vi "Dashboard Main.vi"() -> ()   [LabVIEW 2020]
uses:
  <vilib>/Utility/miscctls.llb/LVRowAndColumnTypeDef.ctl
  <vilib>/event_ctls.llb/eventvkey.ctl
  d97281b5-a6a5-4d38-a890-f2f672331580.vi
  <vilib>/Array/Sort 2D Array - Pop Stack.vi
  <vilib>/Array/Sort 2D Array - Push Stack.vi
  d97281b5-a6a5-4d38-a890-f2f672331580.vi/269d4b3b-47f5-49e3-8884-44851e4dd9d5.vi
  d97281b5-a6a5-4d38-a890-f2f672331580.vi/6d99389c-673d-4efb-bf33-19b32bcf4cf8.vi
  <vilib>/Rock Robotics/WPI/Dashboard/WPI_DashboardLogging Global.vi
  <vilib>/Rock Robotics/Network Tables/NT Read Numeric Array.vi
  <vilib>/Rock Robotics/Network Tables/NT Write Boolean.vi
  <vilib>/Rock Robotics/Network Tables/NT Write Numeric Array.vi
  TitanLib/Lib/TitanLib.lvlib
  <vilib>/gmath/NI_Gmath.lvlib
panel:
  in  "Camera Settings Right":T1={"Frame Rate"=30, "Compression"=30, "Size"=1, "DB Camera Config"=FALSE} {"Frame Rate" scale=1.0..30.0; "Compression" scale=100.0..-1.0; "Size" items=["640x480", "320x240", "160x120"]}
  in  "Camera Name Right":string(combo)="No Camera Selection"
  out "Camera Perf":string
  in  "Camera Settings":T1={"Frame Rate"=30, "Compression"=30, "Size"=1, "DB Camera Config"=FALSE} {"Frame Rate" scale=1.0..30.0; "Compression" scale=100.0..-1.0; "Size" items=["640x480", "320x240", "160x120"]}
  in  "TCP":refnum<k5>
  in  "Rec Mode":enum32{"Stop", "Record", "Playback"}(radio)
  out "Robot IP":string
  out "Image Message":string="Timeout in Camera Communications"
  in  "Dashboard Tab":T2(tab)
  in  "Select Auto":string(combo)="Select Autonomous ..."
  out "NT Connection":bool
  out "MotorChart R":cluster{"Numeric":dbl, "Numeric":dbl}(graph)
  out "MotorChart L":cluster{"Numeric":dbl, "Numeric":dbl}(graph)
  out "MotorSliders R":cluster{"MotorSlide1":dbl, "MotorSlide2":dbl} {"MotorSlide2" scale=-1.0..1.0 scale format="%#_2e"; "MotorSlide1" scale=-1.0..1.0 scale format="%#_2e"}
  out "MotorSliders L":cluster{"MotorSlide1":dbl, "MotorSlide2":dbl} {"MotorSlide2" scale=-1.0..1.0 scale format="%#_2e"; "MotorSlide1" scale=-1.0..1.0 scale format="%#_2e"}
  out "Gyro":dbl(knob) scale=0.0..360.0
  out "JS1 Z":dbl(slide) scale=-1.0..1.0 scale format="%#_2e"
  out "JS1 Graph":cluster{"X":dbl, "Y":dbl}[](graph)
  out "JS1 Buttons":T3
  out "JS2 Z":dbl(slide) scale=-1.0..1.0 scale format="%#_2e"
  out "JS2 Graph":cluster{"X":dbl, "Y":dbl}[](graph)
  out "JS2 Buttons":T3
  out "Mode":T4(ring)=enum."Auto Disabled"
  out "Right Camera Perf":cluster{"Bandwidth (Mbps)":dbl, "FPS":dbl}
  out "Camera Image Right":T5(plugin-control)
  in  "DB/String 9":string
  in  "DB/String 8":string
  in  "DB/String 7":string
  in  "DB/String 6":string
  in  "DB/String 5":string
  in  "DB/String 4":string
  in  "DB/String 3":string
  in  "DB/String 2":string
  in  "DB/String 1":string
  in  "DB/String 0":string
  in  "DB/Slider 0":dbl(slide) scale=0.0..5.0
  in  "DB/Slider 1":dbl(slide) scale=0.0..5.0
  in  "DB/Slider 2":dbl(slide) scale=0.0..5.0
  in  "DB/Slider 3":dbl(slide) scale=0.0..5.0
  out "DB/LED 3":bool
  out "DB/LED 2":bool
  out "DB/LED 1":bool
  out "DB/LED 0":bool
  in  "DB/Button 3":bool
  in  "DB/Button 2":bool
  in  "DB/Button 1":bool
  in  "DB/Button 0":bool caption="New Name"
  in  "Write to NT":bool
  out "XY Graph":cluster{"xi used":dbl[], "yi":dbl[]}[](graph)=[{"xi used"=[117.817, 120.347, 133.458, 133.569, 133.728, 140.097, 140.372, 145.611, 145.622, 148.991, 149.24, 154.505, 154.505, 154.505, 155.962, 156.215, 158.436, 158.631, 158.645, 158.727, 159.752, 165.924, 166.588, 166.604, 166.611, 169.522, 170.238, 173.905, 173.907, 173.917, 174.361, 178.666, 182.023, 182.317, 182.323, 182.33, 182.338, 182.345, 182.345, 183.404, 183.446, 183.451, 184.324, 184.324, 184.693, 184.725, 194.078, 194.078, 197.98, 200.661, 200.661, 219.836], "yi"=[3628.94, 3646.81, 3743.05, 3743.89, 3745.1, 3650.0, 3650.0, 3837.72, 3837.81, 3700.0, 3700.0, 3910.34, 3910.34, 3910.34, 3922.51, 3924.63, 3700.0, 3700.0, 3700.0, 3750.0, 3700.0, 3770.0, 4013.5, 4013.64, 4013.71, 3900.0, 3800.0, 4078.5, 4078.52, 4078.6, 3900.0, 4000.0, 4100.0, 4050.0, 4155.63, 4155.7, 4000.0, 4000.0, 4000.0, 4050.0, 4100.0, 4000.0, 4000.0, 4100.0, 4177.81, 4178.1, 4100.0, 4100.0, 4305.8, 4250.0, 4250.0, 4530.01]}, {"xi used"=[0.0, 5.0, 10.0, 15.0, 20.0, 25.0, 30.0, 35.0, 40.0, 45.0, 50.0, 55.0, 60.0, 65.0, 70.0, 75.0, 80.0, 85.0, 90.0, 95.0, 100.0, 105.0, 110.0, 115.0, 120.0, 125.0, 130.0, 135.0, 140.0, 145.0, 150.0, 155.0, 160.0, 165.0, 170.0, 175.0, 180.0, 185.0, 190.0, 195.0, 200.0, 205.0, 210.0, 215.0, 220.0, 225.0, 230.0, 235.0, 240.0, 245.0], "yi"=[-980.3744808598171, -371.34309861522013, 176.24480259827163, 666.4879484223413, 1103.3572644441058, 1490.6958761946657, 1832.2191091496663, 2131.514488729318, 2392.0417402984467, 2617.1327891663254, 2809.991760586734, 2973.6949797579277, 3111.1909718227503, 3225.3004618685973, 3318.7163749272254, 3394.0038359750674, 3453.6001699330036, 3499.814901666429, 3534.8297559852645, 3560.698657643955, 3579.3477313414537, 3592.575301721237, 3602.051893371288, 3609.3202308241184, 3615.795238556749, 3622.764040990725, 3631.385962492097, 3642.6925273714423, 3657.587459883856, 3676.8466842289404, 3701.1183245508255, 3730.9227049381516, 3766.6523494240782, 3808.571981986281, 3856.8185265469556, 3911.40110697281, 3972.201047075072, 4038.9718706094845, 4111.339301276309, 4188.801262720326, 4270.727878530827, 4356.361472241625, 4444.816567331051, 4535.079887221948, 4626.010355281679, 4716.339094822126, 4804.669429099683, 4889.476881315268, 4969.109174614305, 5041.786232086747]}, {"xi used"=[116.59817122847011, 0.0], "yi"=[117.59817122847011, 5000.0]}]
  in  "Add Cursor":bool
  in  "Delete Cursor":bool
  in  "Interpolation Method":i32(ring)=4 items=["nearest", "linear", "spline", "cubic Hermite", "Lagrange"]
  in  "Static High Goal RPM":dbl
  in  "Use Static Setpoint?":bool
  in  "Test Slider":dbl(slide) scale=0.0..100.0 scale format="%#_3g"
  in  "On/Off":bool caption="Solenoid"
  in  "Test Name":u16(ring) items=["Select the test to run..."]
  in  "Test Tree":string(tree)
  in  "Motor":cluster{"Value":dbl, "Enable":bool} {"Value" scale=-1.0..1.0 scale format="%#_3g"}
  out "Progress":T6 {"Test Progress" scale=0.0..100.0}
  in  "Rev/Fwd":cluster{"Forward":bool, "Reverse":bool}
  in  "Test Ring":u16(ring) items=["Monochrome", "Color"]
  out "Cmd Status":string
  in  "Execute Command":bool
  in  "Command Params":string[][](table)
  in  "Command Selection":i32(listbox)
  in  "CheckList":i32(listbox)
  out "Tree":string(tree)
  out "Camera Image":T5(plugin-control)
  out "Background":bool
  in  "Camera Name":string(combo)="No Camera Selection"
  # "HW"
  # "HW"
  # "Joysticks"
  # "Drive Motors"
  # "Front"
  # "Right"
  # "Left"
  # "Back"
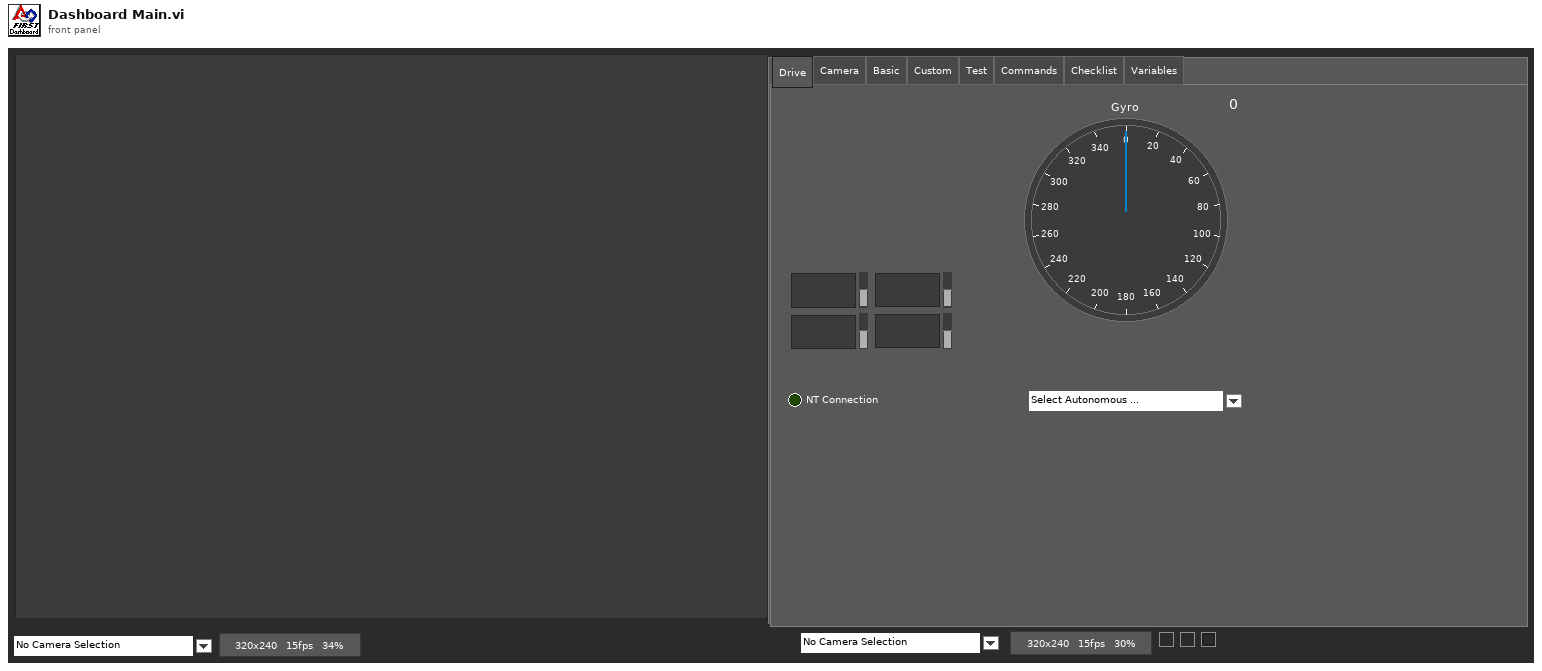
[diagram p1: front panel]
types:
  T1 = cluster{"Frame Rate":i32, "Compression":i32, "Size":u16, "DB Camera Config":bool}
  T2 = enum32{"Drive", "Camera", "Basic", "Custom", "Test", "Commands", "Checklist", "Variables"}
  T3 = cluster{bool, bool, bool, bool, bool, bool, bool, bool, bool, bool, bool, bool}
  T4 = enum8{"Tele-Op Disabled", "Tele-Op Enabled", "Auto Disabled", "Auto Enabled", "Test Disabled", "Test Enabled", "Disconnected", "No Code", "E-Stop"}
  T5 = typedef "IMAQ Image.ctl" = refnum<image>
  T6 = cluster{"Test Progress":u8, "Test Progress Text":string}
  T7 = cluster{"Save Path":path, "Interval (s)":dbl, "Keep":i32}
  T8 = typedef "Image Type" = u32
  T9 = cluster{"IDs":cluster{"RPC field ID":u16, "Unique ID":u16}, "String":string}
  T10 = cluster{"Camera Image":refnum<vi>, "Dashboard Tab":refnum<vi>, "Background":refnum<vi>, "Rec Mode":refnum<vi>, "Test Slider":refnum<vi>, "On/Off ":refnum<vi>, "Test Ring":refnum<vi>, "Rev/Fwd":refnum<vi>, "Test Name":refnum<vi>, "Motor":refnum<vi>, "Progress":refnum<vi>, "CheckList":refnum<vi>, "Tree":refnum<vi>, "Test Tree":refnum<vi>, "Command Params":refnum<vi>, "Command Selection":refnum<vi>, "Execute Command":refnum<vi>, "Cmd Status":refnum<vi>, "Camera Settings":refnum<vi>, "Camera Name":refnum<vi>, "Camera Perf":refnum<vi>, "Camera Settings Right":refnum<vi>, "Camera Name Right":refnum<vi>, "Camera Image Right":refnum<vi>}
  T11 = cluster{"Global Rectangle":i32[], "Contours":cluster{"Contour Type":u32, "ROI Type":u32, "Points":i32[]}[]}
  T12 = cluster{"Camera Name":string, string, "Saved DB Images Info":cluster{"Save Path":path, "Interval (s)":dbl, "Keep":i32}}
  T13 = cluster{"Camera Name Right":string, string, "Saved DB Images Info":cluster{"Save Path":path, "Interval (s)":dbl, "Keep":i32}}
  T14 = cluster{"Operation":enum16{"Update", "Clear"}, "Color Box":u32}[]
  T15 = typedef "eventvkey.ctl" = enum16{"ASCII", "Enter", "Return", "Shift", "Ctrl", "Alt", "Cmd", "Opt", "Caps", "NumLock", "Clear", "Break", "Up", "Down", "Left", "Right", "Insert", "Delete", "Home", "End", "PageUp", "PageDown", "Escape", "Help", "Pause", "ScrollLock", "F1", "F2", "F3", "F4", "F5", "F6", "F7", "F8", "F9", "F10", "F11", "F12", "F13", "F14", "F15", "F16", "F17", "F18", "F19", "F20", "F21", "F22", "F23", "F24", "Play", "VolumeUp", "VolumeDown", "Mute", "Two Byte Char"}
  T16 = cluster{"Image Size":bool, "Image Type":bool, "Pixel Value":bool, "ROI Information":bool, "Zoom Factor":bool}
  T17 = cluster{"Operation":enum16{"Update", "Clear"}, "Color Box":u32}
  T18 = typedef "LVRowAndColumnTypeDef.ctl" = cluster{"Row":i32, "Column":i32}
  T19 = cluster{"Shift":bool, "Ctrl":bool, "Alt":bool, "Cmd":bool, "Opt":bool}
  T20 = cluster{"sorted 2D array":dbl[], "sorted 2D array":dbl[]}
  T21 = cluster{"Name":string, "Color":u32, "Style":u8, "Point Style":u8, "Name Visible":bool, "Allow Drag":bool, "Cursor Mode":u32, "Plot":i32, "Index":i32, "Position":cluster{"X":dbl, "Y":dbl}, "X Scale":u32, "Y Scale":u32, "Watch Plots":i32[], "Watch All Plots":bool, "Plot Area":i32, "Label Offset":cluster{"X":dbl, "Y":dbl}}
  T22 = cluster{"Error Strings":string, "Disable Counts":cluster{u16, u16}, "Rail Faults":cluster{u16, u16, u16}, "Robot IP":string, "DB Mode":u8, "Event Info":cluster{"Name":string, "Type":u8, "Number":u16, "Replay":u8}}
  T23 = cluster{"Storage":cluster{"Disk Free":u64, "RAM Block":u32, "RAM free":u32}, "CPU Utilization":cluster{"CPU % ISR":sgl, "CPU % Time Crit":sgl, "CPU % Timed Str":sgl, "CPU % High":sgl, "CPU % Above":sgl, "CPU % Normal":sgl, "CPU % Low":sgl}, "CAN":cluster{"% Bus Utilization":sgl, "Bus Off Cnt":u32, "TX_FIFO Full Cnt":u32, "Receive Error Cnt":u8, "Transmit Error Cnt":u8}, "HID":cluster{"HID Outputs":u32, "Rumble Low":u16, "Rumble High":u16}[]}
  T24 = cluster{"Status bits":cluster{"Test Mode":bool, "Autonomous":bool, "Enabled":bool, "Code Start":bool, "Brownout":bool, "Reserved 2":bool, "Reserved 3":bool, "E-Stop":bool}, "Code Trace":cluster{"Disabled":bool, "TeleOp":bool, "Auto":bool, "Test":bool}, "Controller Type":enum16{"unknown", "cRIO", "roboRio"}, "Code?":enum16{"unknown", "noCode", "code"}, "Battery V":dbl}
  T25 = cluster{"Control Bits":cluster{"TestMode":bool, "Autonomous":bool, "Enabled":bool, "FMS Present":bool, bool, bool, bool, "E-Stop":bool}, "Team Station ":u8, "Countdown":sgl, "Joystick Values":cluster{"Axes":dbl[], "Buttons":bool[], "POVs":i16[]}[]}
  T26 = cluster{"Axes":dbl[], "Buttons":bool[], "POVs":i16[]}[]
  T27 = cluster{"Axes":dbl[], "Buttons":bool[], "POVs":i16[]}
  T28 = typedef "LVCursorListTypeDef.ctl" = cluster{"Name":string, "Color":u32, "Style":u8, "Point Style":u8, "Name Visible":bool, "Allow Drag":bool, "Cursor Mode":u32, "Plot":i32, "Index":i32, "Position":cluster{"X":dbl, "Y":dbl}, "X Scale":u32, "Y Scale":u32, "Watch Plots":i32[], "Watch All Plots":bool, "Plot Area":i32, "Label Offset":cluster{"X":dbl, "Y":dbl}}[]
  T29 = cluster{"Buttons[0]":bool, "Buttons[1]":bool, "Buttons[2]":bool, "Buttons[3]":bool, "Buttons[4]":bool, "Buttons[5]":bool, "Buttons[6]":bool, "Buttons[7]":bool, "Buttons[8]":bool, "Buttons[9]":bool, "Buttons[10]":bool, "Buttons[11]":bool}
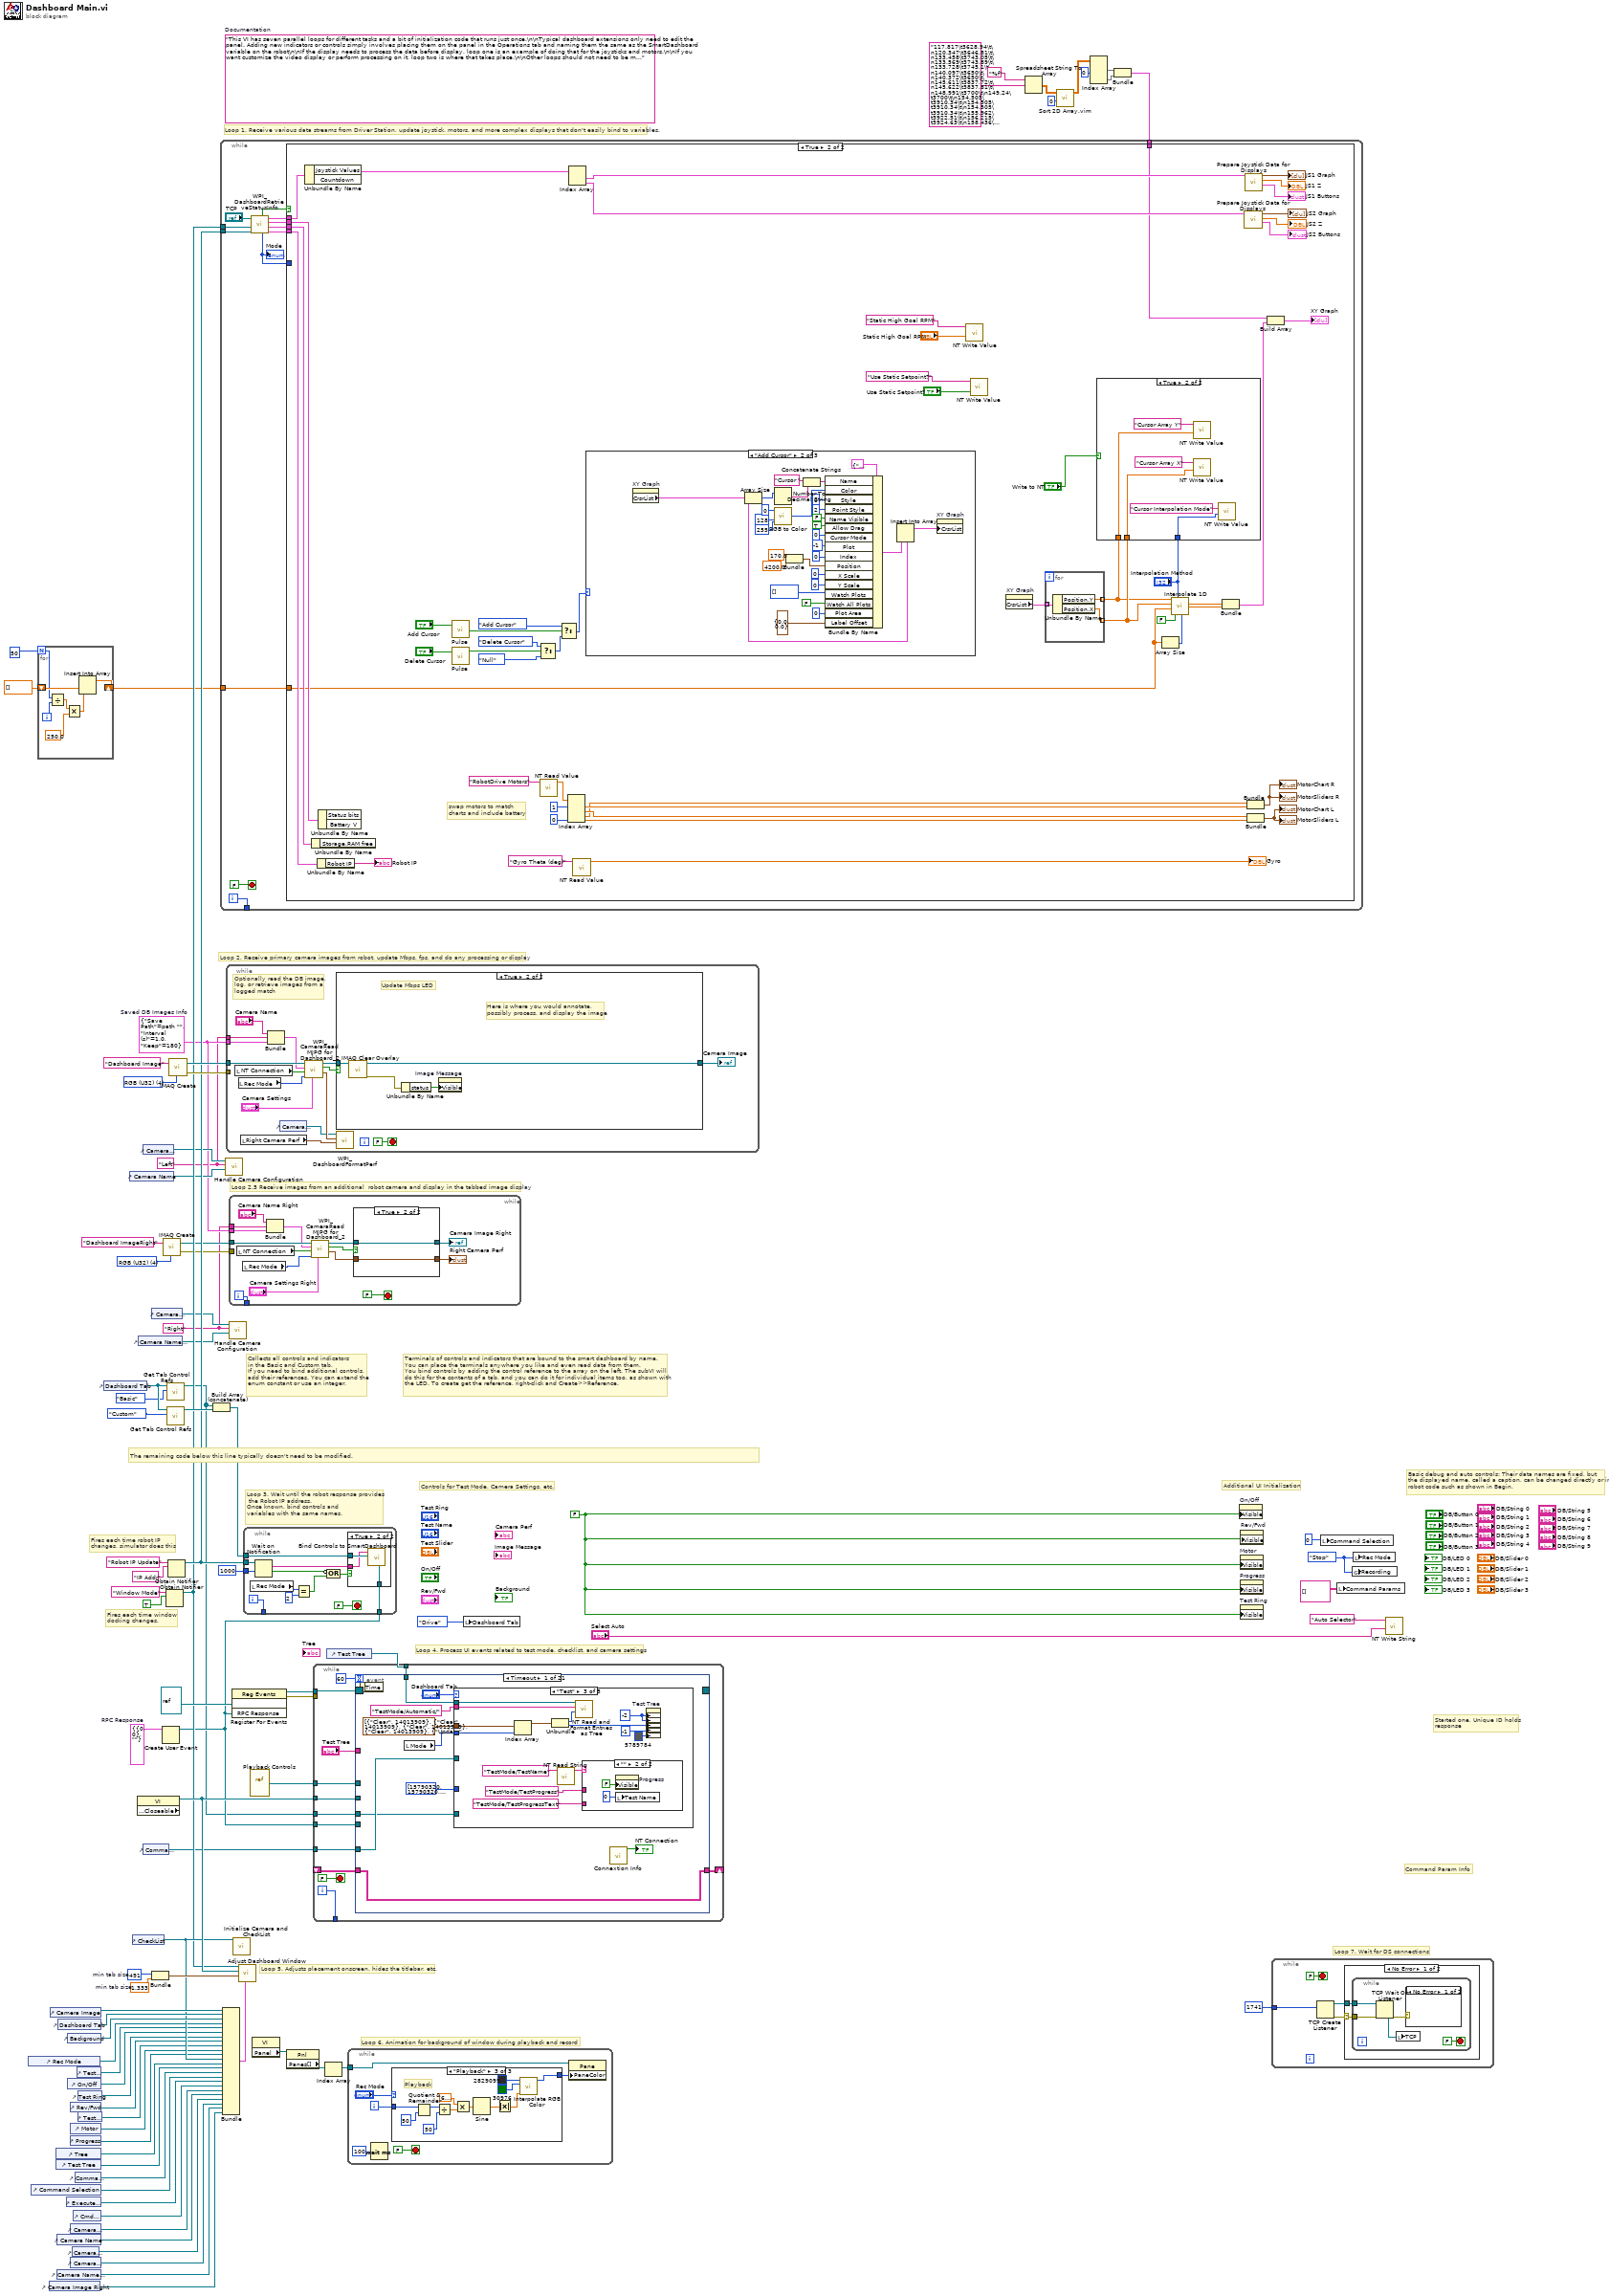
[diagram p0: block diagram]
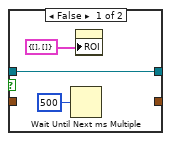
[diagram p2: hidden frame]
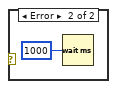
[diagram p3: hidden frame]
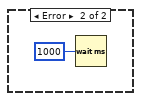
[diagram p4: hidden frame]
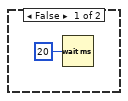
[diagram p5: hidden frame]
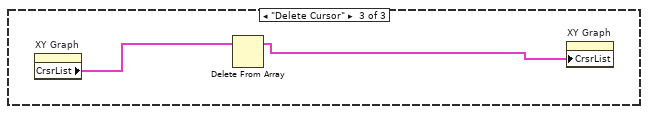
[diagram p8: hidden frame]
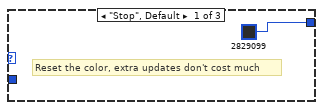
[diagram p9: hidden frame]
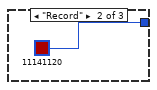
[diagram p10: hidden frame]
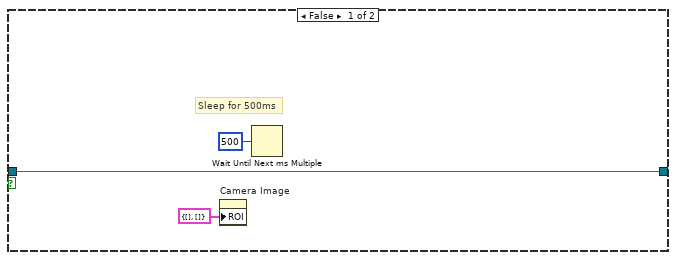
[diagram p12: hidden frame]
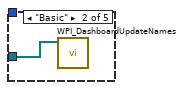
[diagram p14: hidden frame]
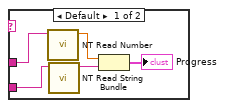
[diagram p15: hidden frame]
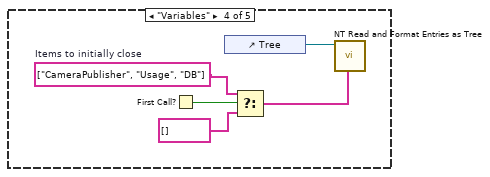
[diagram p16: hidden frame]
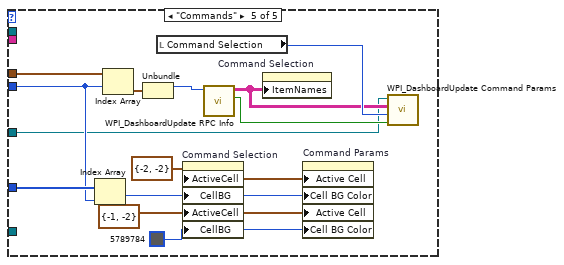
[diagram p17: hidden frame]
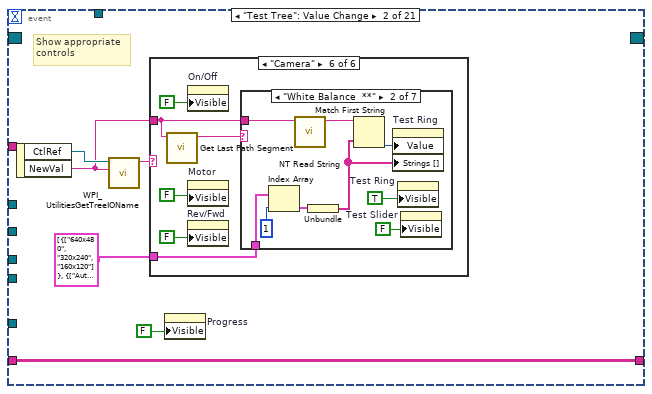
[diagram p18: hidden frame]
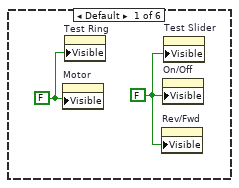
[diagram p19: hidden frame]
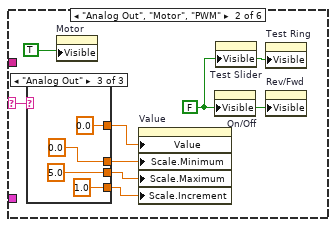
[diagram p20: hidden frame]
diagram:
  w15 = T7 {"Save Path"=path "", "Interval (s)"=1.0, "Keep"=180}  # Saved DB Images Info
  w14 = "Right"
  w13 = "Left"
  w25 = T8 4 items=["Grayscale (U8)", "Grayscale (I16)", "Grayscale (SGL)", "Complex (CSG)", "RGB (U32)", "HSL (U32)", "RGB (U64)"] ("Image Type")
  w41 = T9 {"IDs"={"RPC field ID"=0, "Unique ID"=0}, "String"=""}  # RPC Response
  w64 = 491  # min tab size
  w63 = 1.333  # min tab size
  w71 = enum32{"Stop", "Record", "Playback"}."Stop" ("Rec Mode")
  w48 = FALSE ("Visible")
  (unwired) "This VI has seven parallel loops for different tasks and a bit of initialization code that runs just once.\n\nTypical dashboard extensions only need to edit the panel. Adding new indicators or controls simply involves placing them on the panel in the Operations tab and naming them the same as the SmartDashboard variable on the robot\n\nIf the display needs to process the data before display, loop one is an example of doing that for the joysticks and motors.\n\nIf you want customize the video display or perform processing on it, loop two is where that takes place.\n\nOther loops should not need to be modified. They are pretty standard, and document the task they perform."  # Documentation
  w88 = T8 4 items=["Grayscale (U8)", "Grayscale (I16)", "Grayscale (SGL)", "Complex (CSG)", "RGB (U32)", "HSL (U32)", "RGB (U64)"] ("Image Type")
  # "Loop 2.5 Receive images from an additional  robot camera and display in the tabbed image display"
  # "Command Param Info"
  # "Started one, Unique ID holds\nresponse"
  # "Loop 7. Wait for DS connections"
  # "Basic debug and auto controls: Their data names are fixed, but\nthe displayed name, called a caption, can be changed directly or in\nrobot code such as shown in Begin."
  # "Controls for Test Mode, Camera Settings, etc."
  # "Additional UI Initialization"
  # "Loop 6. Animation for background of window during playback and record"
  # "Fires each time robot IP\nchanges, simulator does this"
  # "Fires each time window\ndocking changes."
  # "Collects all controls and indicators\nin the Basic and Custom tab.\nIf you need to bind additional controls,\nadd their references. You can extend the\nenum constant or use an integer."
  # "The remaining code below this line typically doesn't need to be modified."
  # "Loop 4. Process UI events related to test mode, checklist, and camera settings"
  # "Terminals of controls and indicators that are bound to the smart dashboard by name.\nYou can place the terminals anywhere you like and even read data from them.\nYou bind controls by adding the control reference to the array on the left. The subVI will\ndo this for the contents of a tab, and you can do it for individual items too, as shown with\nthe LED. To create get the reference, right-click and Create>>Reference."
  # "Loop 3. Wait until the robot response provides\n the Robot IP address.\nOnce known, bind controls and\nvariables with the same names."
  # "Loop 5. Adjusts placement onscreen, hides the titlebar, etc."
  # "Loop 1. Receive various data streams from Driver Station, update joystick, motors, and more complex displays that don't easily bind to variables."
  # "Loop 2. Receive primary camera images from robot, update Mbps, fps, and do any processing or display"
  n1 = control-ref of="Rec Mode"() -> (w54:refnum<vi>)
  n2 = control-ref of="Command Selection"() -> (w40:refnum<vi>)
  n3 = for {
    N: 50 ("Graph Points") -> [w93]
    shift-right: [w95] -> w10
    shift-left: dbl[] [] -> [w94]
    i -> [w92]
    n4 = Divide(x=w92, y=w93) -> (x/y=w91:dbl)
    n5 = Multiply(x=w91, y=250.0 ("max point")) -> (x*y=w90:dbl)
    n6 = Insert Into Array(array=w94, new element=w90) -> (w95:dbl[])  [unwired: 1 in]
  }
  n7 = control-ref of="Camera Image Right"() -> (w18:refnum<vi>)
  n8 = control-ref of="Camera Image"() -> (w66:refnum<vi>)
  n9 = control-ref of="Tree"() -> (w58:refnum<vi>)
  n10 = control-ref of="Test Tree"() -> (w57:refnum<vi>)
  n11 = control-ref of="Camera Name"() -> (w31:refnum<vi>)
  n12 = control-ref of="Camera Name Right"() -> (w19:refnum<vi>)
  n13 = control-ref of="Dashboard Tab"() -> (w65:refnum<vi>)
  n14 = control-ref of="Execute Command"() -> (w42:refnum<vi>)
  n15 = control-ref of="Background"() -> (w61:refnum<vi>)
  n16 = control-ref of="On/Off"() -> (w52:refnum<vi>)
  n17 = control-ref of="Progress"() -> (w49:refnum<vi>)
  n18 = control-ref of="Camera Settings"() -> (w32:refnum<vi>)
  n19 = control-ref of="Camera Settings Right"() -> (w20:refnum<vi>)
  n20 = control-ref of="Rev/Fwd"() -> (w50:refnum<vi>)
  n21 = control-ref of="Motor"() -> (w55:refnum<vi>)
  n22 = control-ref of="Camera Perf"() -> (w30:refnum<vi>)
  n23 = control-ref of="Cmd Status"() -> (w36:refnum<vi>)
  n24 = control-ref of="Command Params"() -> (w43:refnum<vi>)
  n25 = control-ref of="Test Slider"() -> (w53:refnum<vi>)
  n26 = control-ref of="Test Ring"() -> (w51:refnum<vi>)
  n27 = control-ref of="Test Name"() -> (w56:refnum<vi>)
  n28 = control-ref of="Dashboard Tab"() -> (w69:refnum<vi>)
  n29 = control-ref of="Camera Name"() -> (w33:refnum<vi>)
  n30 = control-ref of="CheckList"() -> (w59:refnum<vi>)
  n31 = property class="VI" props=["Front Panel.Closeable"]() -> (reference out=w70:refnum<vi>)  [unwired: 2 in, 2 out]
  n32 = control-ref of="Camera Name Right"() -> (w21:refnum<vi>)
  n33 = control-ref of="Camera Settings"() -> (w34:refnum<vi>)
  n34 = control-ref of="Command Params"() -> (w35:refnum<vi>)
  n35 = control-ref of="Camera Settings Right"() -> (w22:refnum<vi>)
  n36 = Bundle("min tab size"=w64, "min tab size"=w63) -> (w62:cluster{"min tab size":i32, "min tab size":dbl})  [unwired: 1 in]
  n37 = Create User Event(user event datatype=w41) -> (user event=w37:refnum<user-event>)  [unwired: 1 in, 1 out]
  n38 = call "IMAQ Create"("Image Name"="Dashboard ImageRight", "Image Type"=w25) -> ("New Image"=w24:T5, "error out"=w23:errorcluster)  [unwired: 2 in, 1 out]
  n39 = Obtain Notifier(name (unnamed)="Window Mode", notification data type=TRUE) -> (notifier out=w46:refnum<notifier>)  [unwired: 2 in, 2 out]
  n40 = call <vilib>:"Get Tab Control Refs.vi"("Page Index"=T2."Basic" ("Dashboard Tab"), "TabControl in"=w69) -> ("ControlsOnPage"=w29:refnum<vi>[])  [unwired: 9 in]
  n41 = call <vilib>:"Get Tab Control Refs.vi"("Page Index"=T2."Custom" ("Dashboard Tab"), "TabControl in"=w69) -> ("ControlsOnPage"=w68:refnum<vi>[])  [unwired: 9 in]
  n42 = Obtain Notifier(name (unnamed)="Robot IP Update", notification data type="IP Addr" ("name (unnamed)")) -> (notifier out=w47:refnum<notifier>)  [unwired: 2 in, 2 out]
  n43 = call "IMAQ Create"("Image Name"="Dashboard Image", "Image Type"=w88) -> ("New Image"=w86:T5, "error out"=w85:errorcluster)  [unwired: 2 in, 1 out]
  n44 = Build Array (concatenate)(w29, w68) -> (w67:refnum<vi>[])
  n45 = Bundle("Camera Image"=w66, "Dashboard Tab"=w65, "Background"=w61, "Rec Mode"=w54, "Test Slider"=w53, "On/Off"=w52, "Test Ring"=w51, "Rev/Fwd"=w50, "Test Name"=w56, "Motor"=w55, "Progress"=w49, "CheckList"=w59, "Tree"=w58, "Test Tree"=w57, "Command Params"=w43, "Command Selection"=w40, "Execute Command"=w42, "Cmd Status"=w36, "Camera Settings"=w32, "Camera Name"=w31, "Camera Perf"=w30, "Camera Settings Right"=w20, "Camera Name Right"=w19, "Camera Image Right"=w18) -> (w60:T10)  [unwired: 1 in]
  n46 = call "Handle Camera Configuration.vi"("CameraNameRef"=w33, "Display Name"=w13, "ClusterRef"=w34) -> ()  [unwired: 9 in]
  n47 = while {
    tunnel: w86 -> [w109]
    tunnel: w85 -> [_]
    tunnel: w15 -> [w102]
    tunnel: w13 -> [w99]
    stop <- FALSE stop-if-true
    # "Optionally read the DB image,\nlog, or retrieve images from a\nlogged match"
    n48 = local read "NT Connection"() -> (w103:bool)
    n49 = local read "Rec Mode"() -> (w106:enum32{"Stop", "Record", "Playback"})
    n50 = local read "Right Camera Perf"() -> (w97:cluster{"Bandwidth (Mbps)":dbl, "FPS":dbl})
    n51 = Bundle("Camera Name"="Camera Name", w99, "Saved DB Images Info"=w102) -> (w101:T12)  [unwired: 1 in]
    n52 = control-ref of="Camera Perf"() -> (w96:refnum<vi>)
    n53 = call <vilib>:"WPI_CameraRead MJPG for Dashboard_2.vi"("Camera Settings"="Camera Settings", "Rec Mode"=w106, "NT Connection"=w103, "Capture Info"=w101, "Image in"=w109) -> ("perf info"=w98:cluster{"Bandwidth (Mbps)":dbl, "fps":dbl}, "Active"=w107:bool, "Image\\ out"=w108:T5)  [unwired: 4 in]
    n54 = case shown="True" w107 {
      tunnel: w108 -> [w112 w115]
      tunnel: [w112 w114] -> w104
      frame False {
        # "Sleep for 500ms"
        n55 = property on="Camera Image" class="ImageControl"("ROI"=T11 {"Global Rectangle"=[], "Contours"=[]}) -> ()  [unwired: 2 in, 2 out]
        n56 = Wait Until Next ms Multiple(millisecond multiple=u32 500) -> ()  [unwired: 1 out]
      }
      frame True {
        # "Here is where you would annotate,\npossibly process, and display the image"
        # "Update Mbps LED"
        n57 = call "IMAQ Clear Overlay"("Image"=w115) -> ("error out"=w116:errorcluster, "Image Out"=w114:T5)  [unwired: 2 in, 7 out]
        n58 = Unbundle By Name(w116) -> ("status"=w117:bool)
        n59 = property on="Image Message" class="Str"("Visible"=w117) -> ()  [unwired: 2 in, 2 out]
      }
    }
    "Camera Image" <- w104
    n60 = call <vilib>:"WPI_DashboardFormatPerf.vi"("Right Camera Perf"=w97, "Performance"=w98, "String in"=w96) -> ()  [unwired: 9 in]
  }
  n61 = call "Handle Camera Configuration.vi"("CameraNameRef"=w21, "Display Name"=w14, "ClusterRef"=w22) -> ()  [unwired: 9 in]
  n62 = while {
    tunnel: w24 -> [w132]
    tunnel: w23 -> [_]
    tunnel: [w127] -> _
    tunnel: w15 -> [w123]
    tunnel: w14 -> [w120]
    i -> [w127]
    stop <- FALSE stop-if-true
    n63 = local read "NT Connection"() -> (w124:bool)
    n64 = local read "Rec Mode"() -> (w131:enum32{"Stop", "Record", "Playback"})
    n65 = Bundle("Camera Name Right"="Camera Name Right", w120, "Saved DB Images Info"=w123) -> (w122:T13)  [unwired: 1 in]
    n66 = call <vilib>:"WPI_CameraRead MJPG for Dashboard_2.vi"("Camera Settings"="Camera Settings Right", "Rec Mode"=w131, "NT Connection"=w124, "Capture Info"=w122, "Image in"=w132) -> ("perf info"=w118:cluster{"Bandwidth (Mbps)":dbl, "fps":dbl}, "Active"=w126:bool, "Image\\ out"=w129:T5)  [unwired: 4 in]
    n67 = case shown="True" w126 {
      tunnel: w129 -> [w134 w137]
      tunnel: [w134 w137] -> w125
      tunnel: [_ w136] -> w119
      tunnel: w118 -> [_ w136]
      frame False {
        n68 = Wait Until Next ms Multiple(millisecond multiple=u32 500) -> ()  [unwired: 1 out]
        n69 = property on="Camera Image Right" class="ImageControl"("ROI"=T11 {"Global Rectangle"=[], "Contours"=[]}) -> ()  [unwired: 2 in, 2 out]
      }
      frame True {
      }
    }
    "Camera Image Right" <- w125
    "Right Camera Perf" <- w119
  }
  n70 = register-events(refnum<vi> refnum, w37) -> (reference out=w75:refnum<event-registration>, error out=w74:errorcluster)  [unwired: 2 in]
  n71 = call "Initialize Camera and CheckList.vi"("ListBox in"=w59) -> ()  [unwired: 11 in]
  n72 = call "Adjust Dashboard Window.vi"("Sizing Refnums"=w60, "Size Constraints"=w62, "VI"=w70, "WIn Mode"=w46) -> ()  [unwired: 8 in]
  n73 = while {
    tunnel: w67 -> [w149]
    tunnel: w47 -> [w147]
    tunnel: [w145] -> _
    tunnel: u32 1000 ("milliseconds to wait") -> [w144]
    tunnel: w37 -> [w138]
    i -> [w145]
    stop <- FALSE stop-if-true
    n74 = local read "Rec Mode"() -> (w140:enum32{"Stop", "Record", "Playback"})
    n75 = Wait on Notification(notifier=w147, timeout in ms (-1)=w144) -> (notification=w146:string, timed out?=w142:bool)  [unwired: 2 in, 2 out]
    n76 = Equal?(x=w140, y=u16 2 ("Rec Mode")) -> (x = y?=w141:bool)
    n77 = Compound Arithmetic op=OR(invert w142, w141) -> (w143:bool)
    n78 = case shown="True" w143 {
      tunnel: w149 -> [_ w152]
      tunnel: w146 -> [_ w151]
      tunnel: w138 -> [_ w150]
      frame False {
      }
      frame True {
        n79 = call <vilib>:"Bind Controls to SmartDashboard.vi"("RPC ref"=w150, "Bound Control Refs"=w152, "Server IP Address"=w151) -> ()  [unwired: 9 in]
      }
    }
  }
  n80 = vi-ref "Playback Controls.vi"() -> (w76:refnum<vi>)
  n81 = property class="VI"() -> ("Panel"=w78:refnum<vi>)  [unwired: 2 in, 2 out]
  n82 = property class="Pnl"(reference=w78) -> ("Panes[]"=w79:refnum<vi>[])  [unwired: 1 in, 2 out]
  n83 = Index Array(array=w79) -> (element=w77:refnum<vi>)  [unwired: 1 in]
  n84 = control-ref of="Test Tree"() -> (w80:refnum<vi>)
  n85 = while {
    tunnel: [w162] -> _
    tunnel: w80 -> [w161]
    tunnel: w76 -> [w160]
    tunnel: w75 -> [w159]
    tunnel: w74 -> [_]
    tunnel: w70 -> [w158]
    tunnel: w37 -> [w157]
    tunnel: w35 -> [w156]
    shift-right: [w155] -> _
    shift-left: _ -> [w154]
    tunnel: w29 -> [w153]
    i -> [w162]
    stop <- FALSE stop-if-true
    n86 = event shown="[0] Timeout" {
      selector: w159 -> [_ _ _ _ _ _ _ _ _ _ _ _ _ _ _ _ _ _ _ _ _]
      dyn-events: [_ _ _ _ _ _ _ _ _ _ _ _ _ _ _ _ w422 _ _ _ _] -> _
      timeout: u32 60 ("milliseconds to wait") -> [_ _ _ _ _ _ _ _ _ _ _ _ _ _ _ _ _ _ _ _ _]
      tunnel: w161 -> [w174 _ _ _ _ _ _ _ _ _ _ _ _ _ _ _ _ _ _ _ _]
      tunnel: "Test Tree" -> [_ _ _ _ _ _ _ _ _ _ _ w389 w397 w399 w403 w411 _ _ _ _ _]
      tunnel: w160 -> [_ _ _ _ _ _ _ _ _ _ _ _ _ _ _ _ w424 _ w442 _ _]
      tunnel: w158 -> [_ _ _ _ _ _ _ _ _ _ _ _ _ _ _ _ w420 _ _ _ _]
      tunnel: w157 -> [_ _ _ _ _ _ _ _ _ _ _ _ _ _ _ _ w418 _ _ _ _]
      tunnel: w156 -> [w169 _ _ _ _ _ w340 _ _ _ _ _ _ _ _ _ _ _ _ _ _]
      tunnel: [w168 w217 w319 w324 w333 w337 w338 w347 w357 w364 w376 w388 w395 w398 w402 w410 w417 w437 w439 w443 w456] -> w155
      tunnel: w154 -> [w168 w217 w319 w324 w333 w337 w338 _ _ w364 w376 w388 w395 w398 w402 w410 w417 w437 w439 w443 w456]
      tunnel: w153 -> [w166 _ _ _ _ _ _ _ _ _ _ _ _ _ _ _ _ _ _ _ _]
      event Timeout {
        n87 = event-data() -> ()  [unwired: 1 in, 1 out]
        n88 = local read "Mode"() -> (w171:T4)
        n89 = case shown="\"Test\"" "Dashboard Tab" {
          tunnel: w174 -> [_ _ w190 _ _]
          tunnel: "TestMode/Automatic/" ("Name Pattern") -> [_ _ w189 _ _]
          tunnel: T14 [{"Operation"=enum."Clear", "Color Box"=14013909}, {"Operation"=enum."Clear", "Color Box"=14013909}, {"Operation"=enum."Clear", "Color Box"=14013909}, {"Operation"=enum."Clear", "Color Box"=14013909}, {"Operation"=enum."Update", "Color Box"=14013909}, {"Operation"=enum."Update", "Color Box"=16777215}, {"Operation"=enum."Clear", "Color Box"=14013909}, {"Operation"=enum."Clear", "Color Box"=14013909}, {"Operation"=enum."Clear", "Color Box"=14013909}] -> [_ _ w182 _ w210]
          tunnel: w171 -> [_ _ w181 _ w209]
          tunnel: u32[] [15790320, 15790320, 15790320, 15790320, 16777215, 16777215, 15790320, 15790320, 15790320] -> [_ _ _ _ w215]
          tunnel: w169 -> [_ _ _ _ w203]
          tunnel: w166 -> [_ w176 _ _ _]
          frame "Custom", Default {
          }
          frame "Basic" {
            n90 = call <vilib>:"WPI_DashboardUpdateNames.vi"("Controls on Tab"=w176) -> ()  [unwired: 11 in]
          }
          frame "Test" {
            w188 = -2 ("Active Item:Row Number")
            n91 = Index Array(array=w182, index=w181) -> (element=w183:T17)
            n92 = Unbundle(w183) -> ("Operation"=w184:enum16{"Update", "Clear"}, "Color Box"=w185:u32)
            n93 = call <vilib>:"NT Read String.vi"("Name"="TestMode/TestName") -> ("String"=w179:string)  [unwired: 9 in, 1 out]
            n94 = call <vilib>:"NT Read and Format Entries as Tree.vi"("Operation"=w184, "Name Pattern"=w189, "Tree Refnum"=w190) -> ()  [unwired: 7 in, 2 out]
            n95 = case shown="\"\"" w179 {
              tunnel: "TestMode/TestProgress" ("Name") -> [w192 _]
              tunnel: "TestMode/TestProgressText" ("Name") -> [w191 _]
              frame Default {
                n96 = call <vilib>:"NT Read Number.vi"("Name"=w192) -> ("Numeric"=w193:dbl)  [unwired: 9 in, 1 out]
                n97 = call <vilib>:"NT Read String.vi"("Name"=w191) -> ("String"=w194:string)  [unwired: 9 in, 1 out]
                n98 = Bundle("Numeric"=w193, "String"=w194) -> (→"Progress":cluster{"Numeric":dbl, "String":string})  [unwired: 1 in]
              }
              frame "" {
                n99 = property on="Progress" class="Clust (strict)"("Visible"=FALSE) -> ()  [unwired: 2 in, 2 out]
                n100 = local write "Test Name"(u16 0) -> ()
              }
            }
            n101 = property on="Test Tree" class="Tree (strict)"("Active Item Row Number"=w188, "ActiveColNum"=w188, "CellBG"=w185, "Active Item Row Number"=-1 ("Active Item:Row Number"), "CellBG"=u32 5789784 ("Color Box")) -> ()  [unwired: 2 in, 2 out]
          }
          frame "Variables" {
            w200 = string[] ["CameraPublisher", "Usage", "DB"]  # Items to initially close
            n102 = First Call?() -> (First Call?: T/F=w201:bool)
            n103 = control-ref of="Tree"() -> (w202:refnum<vi>)
            n104 = Select(t=w200, s=w201, f=string[] []) -> (s? t:f=w198:string[])
            n105 = call <vilib>:"NT Read and Format Entries as Tree.vi"("Tags to  Close"=w198, "Tree Refnum"=w202) -> ()  [unwired: 8 in, 2 out]
          }
          frame "Commands" {
            w211 = u32 5789784 ("Color Box")
            w212 = T18 {"Row"=-1, "Column"=-2} ("Active Cell:Active Cell")
            w214 = T18 {"Row"=-2, "Column"=-2} ("Active Cell:Active Cell")
            n106 = Index Array(array=w215, index=w209) -> (element=w213:u32)
            n107 = Index Array(array=w210, index=w209) -> (element=w208:T17)
            n108 = Unbundle(w208) -> ("Operation"=w207:enum16{"Update", "Clear"})  [unwired: 1 out]
            n109 = local read "Command Selection"() -> (w206:i32)
            n110 = property on="Command Selection" class="MCListbox (strict)"("ActiveCell"=w214, "CellBG"=w213, "ActiveCell"=w212, "CellBG"=w211) -> ()  [unwired: 2 in, 2 out]
            n111 = call <vilib>:"WPI_DashboardUpdate RPC Info.vi"("Operation"=w207) -> ("update"=w205:bool, "commands"=w204:string[][])  [unwired: 9 in]
            n112 = property on="Command Selection" class="MCListbox (strict)"("ItemNames"=w204) -> ()  [unwired: 2 in, 2 out]
            n113 = property on="Command Params" class="Tbl (strict)"("Active Cell"=w214, "Cell BG Color"=w213, "Active Cell"=w212, "Cell BG Color"=w211) -> ()  [unwired: 2 in, 2 out]
            n114 = call <vilib>:"WPI_DashboardUpdate Command Params.vi"("Update"=w205, "NewVal"=w206, "Commands"=w204, "Param Tbl"=w203) -> ()  [unwired: 7 in, 1 out]
          }
        }
        n115 = call <vilib>:"Connextion Info.vi"() -> ("Connected"=→"NT Connection":bool)  [unwired: 10 in, 1 out]
      }
      event "Test Tree": Value Change {
        # "Show appropriate\ncontrols"
        n116 = event-data() -> ("CtlRef"=w220:refnum<vi>, "NewVal"=w218:string)  [unwired: 1 in]
        n117 = call <vilib>:"WPI_UtilitiesGetTreeIOName.vi"("NewVal"=w218, "TreeControl in"=w220) -> ("I/O Name"=w221:string)  [unwired: 9 in]
        n118 = case shown="\"Camera\"" w221 {
          selector: w221 -> [_ w228 _ w250 w259 _]
          tunnel: w218 -> [_ _ w247 w249 _ w266]
          tunnel: cluster{string[]}[] [{["640x480", "320x240", "160x120"]}, {["Auto", "Fixed indoor", "Fixed outdoor 1", "Fixed outdoor 2", "Fixed fluorescent 1", "Fixed fluorescent 2", "Hold current"]}, {["Auto", "Flicker-free 50 Hz", "Flicker-free 60 Hz", "Hold current"]}, {["None", "Prioritize frame rate", "Prioritize image quality"]}, {["Monochrome", "Color"]}] -> [_ _ _ _ _ w265]
          frame Default {
            w223 = FALSE ("Visible")
            w222 = FALSE ("Visible")
            n119 = property on="Motor" class="Clust (strict)"("Visible"=w222) -> ()  [unwired: 2 in, 2 out]
            n120 = property on="Test Ring" class="Ring (strict)"("Visible"=w222) -> ()  [unwired: 2 in, 2 out]
            n121 = property on="Rev/Fwd" class="Clust (strict)"("Visible"=w223) -> ()  [unwired: 2 in, 2 out]
            n122 = property on="On/Off" class="Bool (strict)"("Visible"=w223) -> ()  [unwired: 2 in, 2 out]
            n123 = property on="Test Slider" class="Slide (strict)"("Visible"=w223) -> ()  [unwired: 2 in, 2 out]
          }
          frame "Analog Out", "Motor", "PWM" {
            w229 = FALSE ("Visible")
            n124 = case shown="\"Analog Out\"" w228 {
              tunnel: [1.0 ("Value") -1.0 ("Value") 0.0 ("Value")] -> w227
              tunnel: [255.0 ("Value") 1.0 ("Value") 5.0 ("Value")] -> w226
              tunnel: [128.0 ("Value") 0.0 ("Value") 0.0 ("Value")] -> w225
              tunnel: [64.0 ("Value") 0.5 ("Value") 1.0 ("Value")] -> w224
              frame "PWM" {
              }
              frame "Motor", Default {
              }
              frame "Analog Out" {
              }
            }
            n125 = property on="Motor" class="Clust (strict)"("Visible"=TRUE) -> ()  [unwired: 2 in, 2 out]
            n126 = property on="Value" class="Slide (strict)"("Value"=w225, "Scale.Minimum"=w227, "Scale.Maximum"=w226, "Scale.Increment"=w224) -> ()  [unwired: 2 in, 2 out]
            n127 = property on="On/Off" class="Bool (strict)"("Visible"=w229) -> ()  [unwired: 2 in, 2 out]
            n128 = property on="Test Slider" class="Slide (strict)"("Visible"=w229) -> ()  [unwired: 2 in, 2 out]
            n129 = property on="Test Ring" class="Ring (strict)"("Visible"=w229) -> ()  [unwired: 2 in, 2 out]
            n130 = property on="Rev/Fwd" class="Clust (strict)"("Visible"=w229) -> ()  [unwired: 2 in, 2 out]
          }
          frame "Servo" {
            w245 = FALSE ("Visible")
            n131 = call <vilib>:"NT Read Number.vi"("Name"=w247) -> ("Numeric"=w246:dbl)  [unwired: 9 in, 1 out]
            n132 = property on="Test Slider" class="Slide (strict)"("Visible"=TRUE, "Scale.Maximum"=170.0 ("Scale.Range:Maximum")) -> ()  [unwired: 2 in, 2 out]
            n133 = local write "Test Slider"(w246) -> ()
            n134 = property on="Motor" class="Clust (strict)"("Visible"=w245) -> ()  [unwired: 2 in, 2 out]
            n135 = property on="Rev/Fwd" class="Clust (strict)"("Visible"=w245) -> ()  [unwired: 2 in, 2 out]
            n136 = property on="On/Off" class="Bool (strict)"("Visible"=w245) -> ()  [unwired: 2 in, 2 out]
            n137 = property on="Test Ring" class="Ring (strict)"("Visible"=w245) -> ()  [unwired: 2 in, 2 out]
          }
          frame "Relay", "Solenoid" {
            w248 = FALSE ("Visible")
            n138 = property on="Motor" class="Clust (strict)"("Visible"=w248) -> ()  [unwired: 2 in, 2 out]
            n139 = property on="Test Slider" class="Slide (strict)"("Visible"=w248) -> ()  [unwired: 2 in, 2 out]
            n140 = Search and Replace String(input string=w249, search string="/Value  **", replace string="/Direction") -> (result string=w255:string)  [unwired: 5 in, 3 out]
            n141 = property on="Test Ring" class="Ring (strict)"("Visible"=w248) -> ()  [unwired: 2 in, 2 out]
            n142 = call <vilib>:"NT Read String.vi"("Name"=w255) -> ("String"=w253:string)  [unwired: 9 in, 1 out]
            n143 = Equal?(x="Both directions", y=w253) -> (x = y?=w251:bool)
            n144 = Not(x=w251) -> (.not. x?=w252:bool)
            n145 = property on="Rev/Fwd" class="Clust (strict)"("Visible"=w251) -> ()  [unwired: 2 in, 2 out]
            n146 = property on="On/Off" class="Bool (strict)"("Visible"=w252, "Caption.Text"=w250) -> ()  [unwired: 2 in, 2 out]
          }
          frame "Compressor", "Digital Out" {
            w258 = FALSE ("Visible")
            # "Get direction and finish"
            n147 = property on="Motor" class="Clust (strict)"("Visible"=w258) -> ()  [unwired: 2 in, 2 out]
            n148 = property on="Test Slider" class="Slide (strict)"("Visible"=w258) -> ()  [unwired: 2 in, 2 out]
            n149 = property on="Test Ring" class="Ring (strict)"("Visible"=w258) -> ()  [unwired: 2 in, 2 out]
            n150 = property on="On/Off" class="Bool (strict)"("Visible"=TRUE, "Caption.Text"=w259) -> ()  [unwired: 2 in, 2 out]
            n151 = property on="Rev/Fwd" class="Clust (strict)"("Visible"=FALSE) -> ()  [unwired: 2 in, 2 out]
          }
          frame "Camera" {
            n152 = call <vilib>:"Get Last Path Segment.vi"("String in"=w266) -> ("String out"=w267:string)  [unwired: 10 in]
            n153 = property on="On/Off" class="Bool (strict)"("Visible"=FALSE) -> ()  [unwired: 2 in, 2 out]
            n154 = property on="Motor" class="Clust (strict)"("Visible"=FALSE) -> ()  [unwired: 2 in, 2 out]
            n155 = property on="Rev/Fwd" class="Clust (strict)"("Visible"=FALSE) -> ()  [unwired: 2 in, 2 out]
            n156 = case shown="\"White Balance  **\"" w267 {
              tunnel: w266 -> [w273 w282 w291 w300 w309 _ w315]
              tunnel: w265 -> [w271 w279 w288 w297 w306 _ _]
              frame "Size  **" {
                n157 = Index Array(array=w271) -> (element=w270:cluster{string[]})  [unwired: 1 in]
                n158 = call <vilib>:"NT Read String.vi"("Name"=w273) -> ("String"=w272:string)  [unwired: 9 in, 1 out]
                n159 = Unbundle(w270) -> (w268:string[])
                n160 = Match First String(2:w268, 3:w272) -> (0:w269:i32)  [unwired: 1 out]
                n161 = property on="Test Ring" class="Ring (strict)"("Value"=w269, "Strings []"=w268) -> ()  [unwired: 2 in, 2 out]
                n162 = property on="Test Ring" class="Ring (strict)"("Visible"=TRUE) -> ()  [unwired: 2 in, 2 out]
                n163 = property on="Test Slider" class="Slide (strict)"("Visible"=FALSE) -> ()  [unwired: 2 in, 2 out]
              }
              frame "White Balance  **" {
                n164 = Index Array(array=w279, index=1) -> (element=w280:cluster{string[]})
                n165 = call <vilib>:"NT Read String.vi"("Name"=w282) -> ("String"=w281:string)  [unwired: 9 in, 1 out]
                n166 = Unbundle(w280) -> (w277:string[])
                n167 = Match First String(2:w277, 3:w281) -> (0:w276:i32)  [unwired: 1 out]
                n168 = property on="Test Ring" class="Ring (strict)"("Value"=w276, "Strings []"=w277) -> ()  [unwired: 2 in, 2 out]
                n169 = property on="Test Ring" class="Ring (strict)"("Visible"=TRUE) -> ()  [unwired: 2 in, 2 out]
                n170 = property on="Test Slider" class="Slide (strict)"("Visible"=FALSE) -> ()  [unwired: 2 in, 2 out]
              }
              frame "Exposure  **" {
                n171 = Index Array(array=w288, index=2) -> (element=w289:cluster{string[]})
                n172 = call <vilib>:"NT Read String.vi"("Name"=w291) -> ("String"=w290:string)  [unwired: 9 in, 1 out]
                n173 = Unbundle(w289) -> (w285:string[])
                n174 = Match First String(2:w285, 3:w290) -> (0:w286:i32)  [unwired: 1 out]
                n175 = property on="Test Ring" class="Ring (strict)"("Value"=w286, "Strings []"=w285) -> ()  [unwired: 2 in, 2 out]
                n176 = property on="Test Ring" class="Ring (strict)"("Visible"=TRUE) -> ()  [unwired: 2 in, 2 out]
                n177 = property on="Test Slider" class="Slide (strict)"("Visible"=FALSE) -> ()  [unwired: 2 in, 2 out]
              }
              frame "Exposure Priority  **" {
                n178 = Index Array(array=w297, index=3) -> (element=w298:cluster{string[]})
                n179 = call <vilib>:"NT Read String.vi"("Name"=w300) -> ("String"=w299:string)  [unwired: 9 in, 1 out]
                n180 = Unbundle(w298) -> (w294:string[])
                n181 = Match First String(2:w294, 3:w299) -> (0:w295:i32)  [unwired: 1 out]
                n182 = property on="Test Ring" class="Ring (strict)"("Value"=w295, "Strings []"=w294) -> ()  [unwired: 2 in, 2 out]
                n183 = property on="Test Ring" class="Ring (strict)"("Visible"=TRUE) -> ()  [unwired: 2 in, 2 out]
                n184 = property on="Test Slider" class="Slide (strict)"("Visible"=FALSE) -> ()  [unwired: 2 in, 2 out]
              }
              frame "Color Enable  **" {
                n185 = Index Array(array=w306, index=4) -> (element=w307:cluster{string[]})
                n186 = call <vilib>:"NT Read String.vi"("Name"=w309) -> ("String"=w308:string)  [unwired: 9 in, 1 out]
                n187 = Unbundle(w307) -> (w303:string[])
                n188 = Match First String(2:w303, 3:w308) -> (0:w304:i32)  [unwired: 1 out]
                n189 = property on="Test Ring" class="Ring (strict)"("Value"=w304, "Strings []"=w303) -> ()  [unwired: 2 in, 2 out]
                n190 = property on="Test Ring" class="Ring (strict)"("Visible"=TRUE) -> ()  [unwired: 2 in, 2 out]
                n191 = property on="Test Slider" class="Slide (strict)"("Visible"=FALSE) -> ()  [unwired: 2 in, 2 out]
              }
              frame Default {
                n192 = property on="Test Ring" class="Ring (strict)"("Visible"=FALSE) -> ()  [unwired: 2 in, 2 out]
                n193 = property on="Test Slider" class="Slide (strict)"("Visible"=FALSE) -> ()  [unwired: 2 in, 2 out]
              }
              frame "Brightness  **", "Color Level  **", "Compression  **", "FPS  **", "Sharpness  **" {
                n194 = call <vilib>:"NT Read Number.vi"("Name"=w315) -> ("Numeric"=w314:dbl)  [unwired: 9 in, 1 out]
                n195 = local write "Test Slider"(w314) -> ()
                n196 = property on="Test Slider" class="Slide (strict)"("Visible"=TRUE, "Scale.Maximum"=100.0 ("Scale.Range:Maximum")) -> ()  [unwired: 2 in, 2 out]
                n197 = property on="Test Ring" class="Ring (strict)"("Visible"=FALSE) -> ()  [unwired: 2 in, 2 out]
              }
            }
          }
        }
        n198 = property on="Progress" class="Clust (strict)"("Visible"=FALSE) -> ()  [unwired: 2 in, 2 out]
      }
      event "Test Name": Mouse Enter {
        # "Populate the ring with the list of tests"
        n199 = event-data() -> ()  [unwired: 1 in, 1 out]
        n200 = call <vilib>:"NT Read String Array.vi"("Name"="TestMode/TestList") -> ("String Array"=w323:string[])  [unwired: 9 in, 1 out]
        n201 = Build Array (concatenate)("Select the test to run...", w323) -> (w322:string[])
        n202 = property on="Test Name" class="Ring (strict)"("Strings []"=w322) -> ()  [unwired: 2 in, 2 out]
      }
      event "Test Name": Value Change {
        w325 = FALSE ("Visible")
        # "Tell the robot the test name to run"
        n203 = event-data() -> ("NewVal"=w329:u16)  [unwired: 1 in]
        n204 = property on="Test Name" class="Ring (strict)"() -> ("Strings []"=w330:string[])  [unwired: 2 in, 2 out]
        n205 = local write "Progress"(T6 {"Test Progress"=0, "Test Progress Text"=""} ("Progress")) -> ()
        n206 = Index Array(array=w330, index=w329) -> (element=w328:string)
        n207 = call <vilib>:"NT Write String.vi"("String"=w328, "Name"="TestMode/TestName") -> ()  [unwired: 9 in, 1 out]
        n208 = property on="Progress" class="Clust (strict)"("Visible"=TRUE) -> ()  [unwired: 2 in, 2 out]
        n209 = property on="Motor" class="Clust (strict)"("Visible"=w325) -> ()  [unwired: 2 in, 2 out]
        n210 = property on="Test Slider" class="Slide (strict)"("Visible"=w325) -> ()  [unwired: 2 in, 2 out]
        n211 = property on="On/Off" class="Bool (strict)"("Visible"=w325) -> ()  [unwired: 2 in, 2 out]
        n212 = property on="Rev/Fwd" class="Clust (strict)"("Visible"=w325) -> ()  [unwired: 2 in, 2 out]
        n213 = property on="Test Ring" class="Ring (strict)"("Visible"=w325) -> ()  [unwired: 2 in, 2 out]
      }
      event "Select Auto": Mouse Enter {
        # "Populate the combo box with the list of autonomous options"
        n214 = event-data() -> ()  [unwired: 1 in, 1 out]
        n215 = call <vilib>:"NT Read String Array.vi"("Name"="Auto List") -> ("String Array"=w332:string[])  [unwired: 9 in, 1 out]
        n216 = property on="Select Auto" class="CmbBox"("Strings[]"=w332) -> ()  [unwired: 2 in, 2 out]
      }
      event "Select Auto": Value Change {
        # "User modified the Auto Selection. Write to NT variable so robot knows."
        n217 = event-data() -> ("NewVal"=w335:string)  [unwired: 1 in]
        n218 = call <vilib>:"NT Write String.vi"("String"=w335, "Name"="Auto Selector") -> ()  [unwired: 9 in, 1 out]
      }
      event "Command Selection": Value Change {
        # "Get the params and show in table"
        n219 = event-data() -> ("NewVal"=w341:i32)  [unwired: 1 in]
        n220 = property on="Command Selection" class="MCListbox (strict)"() -> ("ItemNames"=w339:string[][])  [unwired: 2 in, 2 out]
        n221 = call <vilib>:"WPI_DashboardUpdate Command Params.vi"("NewVal"=w341, "Commands"=w339, "Param Tbl"=w340) -> ()  [unwired: 8 in, 1 out]
      }
      event "Execute Command": Value Change {
        # "Started one, Unique ID holds\nresponse"
        n222 = event-data() -> ()  [unwired: 1 in, 1 out]
        n223 = property on="Command Selection" class="MCListbox (strict)"() -> ("ItemNames"=w352:string[][])  [unwired: 2 in, 2 out]
        n224 = Index Array(array=w352, index (row)="Command Selection", index (col)=0) -> (element=w350:string)
        n225 = call <vilib>:"Invoke Commands.vi"("Command Params"="Command Params", "Function Name"=w350) -> ("Params"=w346:u8, "Started"=w345:bool)  [unwired: 7 in, 1 out]
        n226 = Array Subset(array="Command Params", length (row)=w346) -> (w347:string[][])  [unwired: 3 in]
        n227 = Select(t="Executing" ("Cmd Status"), s=w345, f="" ("Cmd Status")) -> (s? t:f=→"Cmd Status":string)
      }
      event "Command Selection": Double Click {
        n228 = event-data() -> ("Row"=w360:i32)  [unwired: 1 in]
        n229 = property on="Command Selection" class="MCListbox (strict)"() -> ("ItemNames"=w363:string[][])  [unwired: 2 in, 2 out]
        n230 = local read "Command Params"() -> (w359:string[][])
        n231 = Index Array(array=w363, index (row)=w360, index (col)=0) -> (element=w361:string)
        n232 = call <vilib>:"Invoke Commands.vi"("Command Params"=w359, "Function Name"=w361) -> ("Params"=w358:u8, "Started"=w353:bool)  [unwired: 7 in, 1 out]
        n233 = Array Subset(array=w359, length (row)=w358) -> (w357:string[][])  [unwired: 3 in]
        n234 = Select(t="Executing" ("Cmd Status"), s=w353, f="" ("Cmd Status")) -> (s? t:f=w354:string)
        n235 = local write "Cmd Status"(w354) -> ()
      }
      event "CheckList": Double Click {
        # "Shift clears all"
        # "Update symbols on the listbox"
        n236 = event-data() -> ("PlatMods.Shift"=w365:bool, "Row"=w367:i32)  [unwired: 1 in]
        n237 = case shown="True" w365 {
          tunnel: w367 -> [w371 _]
          tunnel: 1 -> [w370 _]
          frame False {
            n238 = property on="CheckList" class="LstBox (strict)"() -> ("Item Symbols"=w369:i32[])  [unwired: 2 in, 2 out]
            n239 = Replace Array Subset(array=w369, new element=w370, index=w371) -> (w368:i32[])
            n240 = property on="CheckList" class="LstBox (strict)"("Item Symbols"=w368) -> ()  [unwired: 2 in, 2 out]
          }
          frame True {
            w372 = 0 ("Top Row")
            n241 = property on="CheckList" class="LstBox (strict)"() -> ("Number of Rows"=w374:u32)  [unwired: 2 in, 2 out]
            n242 = Initialize Array(0, w374) -> (w373:i32[])
            n243 = property on="CheckList" class="LstBox (strict)"("Top Row"=w372, "Value"=w372, "Item Symbols"=w373) -> ()  [unwired: 2 in, 2 out]
          }
        }
      }
      event "CheckList": Key Down {
        # "Update symbols on the listbox\nLeft and right keys check and uncheck"
        n244 = event-data() -> ("VKey"=w378:T15)  [unwired: 1 in]
        n245 = case shown="\"Left\", \"Right\"" w378 {
          selector: w378 -> [w383 _]
          tunnel: eventvkey."Left" ("VKey") -> [w381 _]
          frame "Left", "Right" {
            n246 = Equal?(x=w381, y=w383) -> (x = y?=w382:bool)
            n247 = Select(t=0, s=w382, f=1) -> (s? t:f=w384:i32)
            n248 = property on="CheckList" class="LstBox (strict)"() -> ("Item Symbols"=w387:i32[])  [unwired: 2 in, 2 out]
            n249 = Replace Array Subset(array=w387, new element=w384, index="CheckList") -> (w386:i32[])
            n250 = property on="CheckList" class="LstBox (strict)"("Item Symbols"=w386) -> ()  [unwired: 2 in, 2 out]
          }
          frame Default {
          }
        }
      }
      event "Motor.Enable": Value Change {
        # "When the test mode otor enable helper is set, update that\ntree row item's value"
        n251 = event-data() -> ("NewVal"=w393:bool)  [unwired: 1 in]
        n252 = Unbundle("Motor") -> ("Value"=w392:dbl)  [unwired: 1 out]
        n253 = Select(t=w392, s=w393, f=0.0) -> (s? t:f=w390:dbl)
        n254 = call <vilib>:"NT Write Number.vi"("Numeric"=w390, "Name"=w389) -> ()  [unwired: 9 in, 1 out]
      }
      event "Test Slider": Value Change {
        # "When the test mode slider helper is set, update that\ntree row item's value"
        n255 = event-data() -> ("NewVal"=w396:dbl)  [unwired: 1 in]
        n256 = call <vilib>:"NT Write Number.vi"("Numeric"=w396, "Name"=w397) -> ()  [unwired: 9 in, 1 out]
      }
      event "On/Off": Value Change {
        # "When the test mode on/off helper value is set, update that\ntree row item's value"
        n257 = event-data() -> ("NewVal"=w401:bool)  [unwired: 1 in]
        n258 = Boolean To (0,1)(Boolean=w401) -> (0, 1=w400:i16)
        n259 = call <vilib>:"NT Write Number.vi"("Numeric"=w400, "Name"=w399) -> ()  [unwired: 9 in, 1 out]
      }
      event "Rev/Fwd": Value Change {
        # "When the test mode helper value for relays is set, update that\ntree row item's value"
        n260 = event-data() -> ("NewVal.Forward"=w409:bool, "NewVal.Reverse"=w408:bool)  [unwired: 1 in]
        n261 = Boolean To (0,1)(Boolean=w409) -> (0, 1=w405:i16)
        n262 = Boolean To (0,1)(Boolean=w408) -> (0, 1=w407:i16)
        n263 = Negate(x=w407) -> (-x=w406:i16)
        n264 = Add(x=w405, y=w406) -> (x+y=w404:i16)
        n265 = call <vilib>:"NT Write Number.vi"("Numeric"=w404, "Name"=w403) -> ()  [unwired: 9 in, 1 out]
      }
      event "Test Ring": Value Change {
        # "When a test mode helper value is selected from the ring,\nset the tree item's variable to the string value"
        n266 = event-data() -> ("NewVal"=w413:u16)  [unwired: 1 in]
        n267 = property on="Test Ring" class="Ring (strict)"() -> ("Strings []"=w414:string[])  [unwired: 2 in, 2 out]
        n268 = Index Array(array=w414, index=w413) -> (element=w412:string)
        n269 = call <vilib>:"NT Write String.vi"("String"=w412, "Name"=w411) -> ()  [unwired: 9 in, 1 out]
      }
      event "Rec Mode": Value Change {
        # "Update globals for recording mode and path to read log from.\nClear when logging and let NetworkTables set path for vision to\nuse."
        n270 = event-data() -> ("NewVal"=w425:enum32{"Stop", "Record", "Playback"})  [unwired: 1 in]
        n271 = global write "WPI_DashboardLogging Global.vi" "Logging Filename"(path "") -> ()
        n272 = global write "WPI_DashboardLogging Global.vi" "Recording"(w425) -> ()
        n273 = case shown="\"Playback\"" w425 {
          tunnel: w424 -> [_ w427 w436]
          tunnel: [_ _ w435] -> w422
          tunnel: [_ _ w434] -> _
          tunnel: w420 -> [_ _ w432]
          tunnel: cluster{i32, i32} {-250, 170} -> [_ _ w431]
          tunnel: [_ _ T16 {"Image Size"=TRUE, "Image Type"=TRUE, "Pixel Value"=TRUE, "ROI Information"=TRUE, "Zoom Factor"=FALSE} ("Image Information Shown:All Elements")] -> w415
          tunnel: [_ _ TRUE ("Zoom Factor")] -> w416
          tunnel: w418 -> [_ _ w428]
          frame Default {
          }
          frame "Stop", "Record" {
            # "Place Window too"
            n274 = invoke class="VI" method="FP.Close"(reference=w427) -> (reference out=w426:refnum<vi>)  [unwired: 2 in, 2 out]
            n275 = invoke class="VI" method="Abort VI"(reference=w426) -> ()  [unwired: 2 in, 3 out]
          }
          frame "Playback" {
            n276 = call "Open Playback Panel.vi"("Offset"=w431, "DB VI Ref"=w432, "Playback in"=w436) -> ("Playback out"=w433:refnum<vi>)  [unwired: 8 in]
            n277 = register-events(w433, w428) -> (reference out=w435:refnum<event-registration>, error out=w434:errorcluster)  [unwired: 2 in]
          }
        }
        n278 = property on="Camera Image Right" class="ImageControl"("Image Information Shown"=w415, "Image Information Visible"=w416) -> ()  [unwired: 2 in, 2 out]
        n279 = property on="Camera Image" class="ImageControl"("Image Information Shown"=w415, "Image Information Visible"=w416) -> ()  [unwired: 2 in, 2 out]
        n280 = call <vilib>:"WPI_DashboardNT Log FieldName Cache.vi"("Operation"=enum16{"Lookup/Add", "Index", "Clear"}."Clear") -> ()  [unwired: 8 in, 3 out]
      }
      event Panel Close {
        w438 = enum32{"Stop", "Record", "Playback"}."Stop" ("Rec Mode")
        # "Playback window has been closed, abort"
        n281 = event-data() -> ()  [unwired: 1 in, 4 out]
        n282 = local write "Rec Mode"(w438) -> ()
        n283 = global write "WPI_DashboardLogging Global.vi" "Recording"(w438) -> ()
      }
      event Panel Close {
        # "Abort playback window and ourself"
        n284 = event-data() -> ()  [unwired: 1 in, 4 out]
        n285 = invoke class="VI" method="FP.Close"(reference=w442) -> (reference out=w441:refnum<vi>)  [unwired: 2 in, 2 out]
        n286 = invoke class="VI" method="Abort VI"(reference=w441) -> (error out=w440:errorcluster)  [unwired: 2 in, 2 out]
        n287 = invoke class="VI" method="Abort VI"(error in=w440) -> ()  [unwired: 2 in, 3 out]
      }
      event User Event {
        n288 = event-data() -> ("IDs"=w449:cluster{"RPC field ID":u16, "Unique ID":u16}, "String"=w448:string)  [unwired: 1 in]
        n289 = Bundle("IDs"=w449, "String"=w448) -> (w447:T9)  [unwired: 1 in]
        n290 = call <vilib>:"Retrieve RPC Response.vi"("RPC Response"=w447) -> ("Output"=w445:string[][])  [unwired: 10 in]
        n291 = Build Array (concatenate)(w443, w445) -> (w444:string[][])
        n292 = local write "Command Params"(w444) -> ()
        n293 = local write "Cmd Status"("" ("Cmd Status")) -> ()
      }
      event "Tree": Double Click {
        n294 = event-data() -> ("PlatMods"=w455:T19, "Tag"=w452:string)  [unwired: 1 in]
        n295 = Unbundle(w455) -> ("Shift"=w454:bool)  [unwired: 4 out]
        n296 = String Subset(string=w452, length (rest)=1 ("length (rest)")) -> (substring=w451:string)  [unwired: 1 in]
        n297 = Not(x=w454) -> (.not. x?=w453:bool)
        n298 = case shown="\"/\"" w451 {
          tunnel: w452 -> [_ w458]
          tunnel: w453 -> [_ w457]
          frame Default {
          }
          frame "/" {
            n299 = call <vilib>:"NT Update Persistence.vi"("Persistence"=w457, "Name"=w458) -> ()  [unwired: 9 in, 1 out]
          }
        }
      }
    }
  }
  n300 = while {
    tunnel: w77 -> [w460]
    i -> [w463]
    stop <- FALSE stop-if-true
    n301 = Wait (ms)(milliseconds to wait=u32 100) -> ()  [unwired: 1 out]
    n302 = case shown="\"Playback\"" "Rec Mode" {
      tunnel: w463 -> [_ _ w478]
      tunnel: [u32 2829099 ("Base Color") u32 11141120 ("Target Color") w467] -> w459
      frame "Stop", Default {
        # "Reset the color, extra updates don't cost much"
      }
      frame "Record" {
      }
      frame "Playback" {
        # "Playback"
        n303 = Quotient & Remainder(x=w478, y=u32 50 ("milliseconds to wait")) -> (x-y*floor(x/y)=w474:u32)  [unwired: 1 out]
        n304 = Divide(x=w474, y=u32 50 ("milliseconds to wait")) -> (x/y=w471:dbl)
        n305 = Multiply(x=6.283185307179586, y=w471) -> (x*y=w476:dbl)
        n306 = Sine(x=w476) -> (sin(x)=w475:dbl)
        n307 = Absolute Value(x=w475) -> (abs(x)=w468:dbl)
        n308 = call "Interpolate RGB Color.vi"("Proportion"=w468, "Target Color"=u32 30976, "Base Color"=u32 2829099) -> ("Result Color"=w467:u32)  [unwired: 8 in]
      }
    }
    n309 = property class="Pane"(reference=w460, "PaneColor"=w459) -> ()  [unwired: 1 in, 2 out]
  }
  n310 = local write "Dashboard Tab"(T2."Drive" ("Dashboard Tab")) -> ()
  n311 = Spreadsheet String To Array(format string="%f", spreadsheet string="117.817\t3628.94\t\n120.347\t3646.81\t\n133.458\t3743.05\t\n133.569\t3743.89\t\n133.728\t3745.1\t\n140.097\t3650\t\n140.372\t3650\t\n145.611\t3837.72\t\n145.622\t3837.81\t\n148.991\t3700\t\n149.24\t3700\t\n154.505\t3910.34\t\n154.505\t3910.34\t\n154.505\t3910.34\t\n155.962\t3922.51\t\n156.215\t3924.63\t\n158.436\t3700\t\n158.631\t3700\t\n158.645\t3700\t\n158.727\t3750\t\n159.752\t3700\t\n165.924\t3770\t\n166.588\t4013.5\t\n166.604\t4013.64\t\n166.611\t4013.71\t\n169.522\t3900\t\n170.238\t3800\t\n173.905\t4078.5\t\n173.907\t4078.52\t\n173.917\t4078.6\t\n174.361\t3900\t\n178.666\t4000\t\n182.023\t4100\t\n182.317\t4050\t\n182.323\t4155.63\t\n182.33\t4155.7\t\n182.338\t4000\t\n182.345\t4000\t\n182.345\t4000\t\n183.404\t4050\t\n183.446\t4100\t\n183.451\t4000\t\n184.324\t4000\t\n184.324\t4100\t\n184.693\t4177.81\t\n184.725\t4178.1\t\n194.078\t4100\t\n194.078\t4100\t\n197.98\t4305.8\t\n200.661\t4250\t\n200.661\t4250\t\n219.836\t4530.01\t\n\t") -> (array=w9:dbl[][])  [unwired: 2 in]
  n312 = call "Sort 2D Array.vim"("index"=0, "2D array"=w9) -> ("sorted 2D array"=w8:dbl[][])  [unwired: 8 in, 1 out]
  n313 = Index Array(array=w8, index (col) #1=0 ("disabled index (col)")) -> (element #1=w6:dbl[], element #2=w7:dbl[])  [unwired: 3 in]
  n314 = Bundle("sorted 2D array"=w6, "sorted 2D array"=w7) -> (w1:T20)  [unwired: 1 in]
  n315 = while {
    tunnel: [w490] -> _
    tunnel: w47 -> [w484]
    tunnel: w46 -> [w481]
    tunnel: w10 -> [w480]
    tunnel: w1 -> [w479]
    i -> [w490]
    stop <- FALSE stop-if-true
    n316 = call <vilib>:"WPI_DashboardRetrieveStatusInfo.vi"("Binding Refnum"=w484, "Window Mode Notifier"=w481, "TCP Cnx"="TCP") -> ("Power and Errors"=w485:T22, "Robot Metrics"=w488:T23, "Status Info"=w489:T24, "Control Info"=w486:T25, "Robot Mode"=w483:T4, "Process?"=w487:bool)  [unwired: 3 in]
    "Mode" <- w483
    n317 = case shown="True" w487 {
      tunnel: w489 -> [_ w544]
      tunnel: w488 -> [_ w543]
      tunnel: w486 -> [_ w542]
      tunnel: w485 -> [_ w541]
      tunnel: w483 -> [_ _]
      tunnel: w480 -> [_ w509]
      tunnel: w479 -> [_ w507]
      frame False {
        n318 = Wait (ms)(milliseconds to wait=u32 20) -> ()  [unwired: 1 out]
      }
      frame True {
        # "swap motors to match\ncharts and include battery"
        n319 = Unbundle By Name(w542) -> ("Joystick Values"=w532:T26)  [unwired: 1 out]
        n320 = Unbundle By Name(w543) -> ()  [unwired: 1 out]
        n321 = Unbundle By Name(w541) -> ("Robot IP"=→"Robot IP":string)
        n322 = Unbundle By Name(w544) -> ()  [unwired: 2 out]
        n323 = call "Pulse.vi"("Input"="Add Cursor") -> ("Output"=w515:bool)  [unwired: 10 in]
        n324 = call "Pulse.vi"("Input"="Delete Cursor") -> ("Output"=w516:bool)  [unwired: 10 in]
        n325 = Select(t=enum16{"Null", "Add Cursor", "Delete Cursor"}."Delete Cursor", s=w516, f=enum16{"Null", "Add Cursor", "Delete Cursor"}."Null") -> (s? t:f=w512:enum16{"Null", "Add Cursor", "Delete Cursor"})
        n326 = call-poly <vilib>:"NT Read Value.vi"("Name"="RobotDrive Motors") -> ("Numeric Array"=w522:dbl[])  [unwired: 9 in, 1 out]
        n327 = Select(t=enum16{"Null", "Add Cursor", "Delete Cursor"}."Add Cursor", s=w515, f=w512) -> (s? t:f=w510:enum16{"Null", "Add Cursor", "Delete Cursor"})
        n328 = Index Array(array=w522, index #1=1, index #4=0) -> (element #1=w536:dbl, element #2=w537:dbl, element #3=w535:dbl, element #4=w540:dbl)  [unwired: 2 in]
        n329 = Index Array(array=w532) -> (element #1=w531:T27, element #2=w527:T27)  [unwired: 2 in]
        n330 = call-poly <vilib>:"NT Read Value.vi"("Name"="Gyro Theta (deg)") -> ("Numeric"=→"Gyro":dbl)  [unwired: 9 in, 1 out]
        n331 = case shown="\"Add Cursor\"" w510 {
          frame "Null", Default {
          }
          frame "Add Cursor" {
            n332 = property on="XY Graph" class="XYGraph (strict)"() -> ("CrsrList"=w555:T28)  [unwired: 2 in, 2 out]
            n333 = Array Size(array=w555) -> (size(s)=w559:i32)
            n334 = Number To Decimal String(number=w559) -> (decimal integer string=w579:string)  [unwired: 1 in]
            n335 = call <vilib>:"RGB to Color.vi"("B"=u8 255, "G"=u8 128, "R"=u8 0) -> ("Color"=w577:u32)
            n336 = Bundle(170.0, 4200.0) -> (w560:cluster{dbl, dbl})  [unwired: 1 in]
            n337 = Concatenate Strings("Cursor ", w579) -> (w578:string)
            n338 = Bundle By Name(cluster=T21 {"Name"="", "Color"=33023, "Style"=0, "Point Style"=0, "Name Visible"=FALSE, "Allow Drag"=FALSE, "Cursor Mode"=0, "Plot"=0, "Index"=0, "Position"={"X"=0.0, "Y"=0.0}, "X Scale"=0, "Y Scale"=0, "Watch Plots"=[], "Watch All Plots"=FALSE, "Plot Area"=0, "Label Offset"={"X"=0.0, "Y"=0.0}} ("Cursor List"), "Name"=w578, "Color"=w577, "Style"=u8 0, "Point Style"=u8 2, "Name Visible"=FALSE, "Allow Drag"=TRUE, "Cursor Mode"=u32 0, "Plot"=-1, "Index"=0, "Position"=w560, "X Scale"=u32 0, "Y Scale"=u32 0, "Watch Plots"=i32[] [], "Watch All Plots"=FALSE, "Plot Area"=0, "Label Offset"=cluster{"X":dbl, "Y":dbl} {"X"=0.0, "Y"=0.0}) -> (w581:T21)
            n339 = Insert Into Array(array=w555, new element=w581) -> (w554:T28)  [unwired: 1 in]
            n340 = property on="XY Graph" class="XYGraph (strict)"("CrsrList"=w554) -> ()  [unwired: 2 in, 2 out]
          }
          frame "Delete Cursor" {
            n341 = property on="XY Graph" class="XYGraph (strict)"() -> ("CrsrList"=w583:T28)  [unwired: 2 in, 2 out]
            n342 = Delete From Array(array=w583) -> (array with subset deleted=w582:T28)  [unwired: 2 in, 1 out]
            n343 = property on="XY Graph" class="XYGraph (strict)"("CrsrList"=w582) -> ()  [unwired: 2 in, 2 out]
          }
        }
        n344 = call-poly <vilib>:"NT Write Value.vi"("Numeric"="Static High Goal RPM", "Name"="Static High Goal RPM") -> ()  [unwired: 9 in, 1 out]
        n345 = call-poly <vilib>:"NT Write Value.vi"("Boolean"="Use Static Setpoint?", "Name"="Use Static Setpoint?") -> ()  [unwired: 9 in, 1 out]
        n346 = property on="XY Graph" class="XYGraph (strict)"() -> ("CrsrList"=w501:T28)  [unwired: 2 in, 2 out]
        n347 = for {
          tunnel: w501 -> [w553] mode=indexing
          tunnel: [w552] -> w498 mode=indexing
          tunnel: [w551] -> w499 mode=indexing
          n348 = Unbundle By Name(w553) -> ("Position.Y"=w552:dbl, "Position.X"=w551:dbl)
        }
        n349 = case shown="True" "Write to NT" {
          tunnel: "Interpolation Method" -> [_ w547]
          tunnel: w499 -> [_ w546]
          tunnel: w498 -> [_ w545]
          frame False {
          }
          frame True {
            n350 = call-poly <vilib>:"NT Write Value.vi"("Numeric Array"=w545, "Name"="Cursor Array Y") -> ()  [unwired: 9 in, 1 out]
            n351 = call-poly <vilib>:"NT Write Value.vi"("Numeric Array"=w546, "Name"="Cursor Array X") -> ()  [unwired: 9 in, 1 out]
            n352 = call-poly <vilib>:"NT Write Value.vi"("Numeric"=w547, "Name"="Cursor Interpolation Mode") -> ()  [unwired: 9 in, 1 out]
          }
        }
        n353 = Array Size(array=w509) -> (size(s)=w504:i32)
        n354 = call <vilib>:"Interpolate 1D.vi"("ntimes"=w504, "method"="Interpolation Method", "X is monotonic"=FALSE, "xi"=w509, "X"=w499, "Y"=w498) -> ("xi used"=w503:dbl[], "yi"=w502:dbl[])  [unwired: 3 in, 1 out]
        n355 = Bundle("xi used"=w503, "yi"=w502) -> (w506:cluster{"xi used":dbl[], "yi":dbl[]})  [unwired: 1 in]
        n356 = call "Prepare Joystick Data for Displays.vi"("Joystick Values"=w527) -> ("Buttons"=→"JS2 Buttons":T29, "Z Axis"=→"JS2 Z":dbl, "Cartesian Data"=→"JS2 Graph":cluster{"X axis":dbl, "X axis":dbl}[])  [unwired: 8 in]
        n357 = call "Prepare Joystick Data for Displays.vi"("Joystick Values"=w531) -> ("Buttons"=→"JS1 Buttons":T29, "Z Axis"=→"JS1 Z":dbl, "Cartesian Data"=→"JS1 Graph":cluster{"X axis":dbl, "X axis":dbl}[])  [unwired: 8 in]
        n358 = Bundle("Numeric"=w535, "Numeric"=w536) -> (→"MotorChart R" →"MotorSliders R":cluster{"Numeric":dbl, "Numeric":dbl})  [unwired: 1 in]
        n359 = Bundle("Numeric"=w537, "Numeric"=w540) -> (→"MotorChart L" →"MotorSliders L":cluster{"Numeric":dbl, "Numeric":dbl})  [unwired: 1 in]
        n360 = Build Array(w507, w506) -> (→"XY Graph":cluster{"xi used":dbl[], "yi":dbl[]}[])
      }
    }
  }
  n361 = property on="On/Off" class="Bool (strict)"("Visible"=w48) -> ()  [unwired: 2 in, 2 out]
  n362 = property on="Motor" class="Clust (strict)"("Visible"=w48) -> ()  [unwired: 2 in, 2 out]
  n363 = property on="Progress" class="Clust (strict)"("Visible"=w48) -> ()  [unwired: 2 in, 2 out]
  n364 = property on="Test Ring" class="Ring (strict)"("Visible"=w48) -> ()  [unwired: 2 in, 2 out]
  n365 = property on="Rev/Fwd" class="Clust (strict)"("Visible"=w48) -> ()  [unwired: 2 in, 2 out]
  n366 = while {
    tunnel: u16 1741 ("timeout ms (25000)") -> [w585]
    stop <- FALSE stop-if-true
    n367 = TCP Create Listener(10:w585) -> (0:w584:errorcluster, 3:w586:refnum<k5>)  [unwired: 4 in, 1 out]
    n368 = case shown="No Error" w584 {
      selector: w584 -> [w588 _]
      tunnel: w586 -> [w589 _]
      frame No Error {
        n369 = while {
          tunnel: w589 -> [w592]
          tunnel: w588 -> [w591]
          stop <- FALSE stop-if-true
          n370 = TCP Wait On Listener(8:w591, 11:w592) -> (0:w593:errorcluster, 4:w594:refnum<k5>)  [unwired: 2 in, 3 out]
          n371 = local write "TCP"(w594) -> ()
          n372 = case shown="No Error" w593 {
            frame No Error {
            }
            frame Error {
              n373 = Wait (ms)(milliseconds to wait=u32 1000) -> ()  [unwired: 1 out]
            }
          }
        }
      }
      frame Error {
        n374 = Wait (ms)(milliseconds to wait=u32 1000) -> ()  [unwired: 1 out]
      }
    }
  }
  n375 = local write "Command Selection"(u16 0 ("milliseconds to wait")) -> ()
  n376 = local write "Command Params"(string[][] [] ("Command Params")) -> ()
  n377 = global write "WPI_DashboardLogging Global.vi" "Recording"(w71) -> ()
  n378 = local write "Rec Mode"(w71) -> ()
  n379 = call <vilib>:"NT Write String.vi"("String"="Select Auto", "Name"="Auto Selector") -> ()  [unwired: 9 in, 1 out]
